vi "ScrollDataChange.vi"(0 "Actual Data":T1[](array[typedef]), 5 "Display Data":T1[](array[typedef]), 9 "Bounds  Of Picture":T3, 11 "Delta":i32) -> (4 "Actual Dataout":T1[](array[typedef]), 6 "Display Data out":T1[](array[typedef]), 8 "ScrollChange?":bool)   [LabVIEW 2014, in "SmartPalette.lvlib"]
uses:
  SmartPalette.lvlib
  Controls/Palette Data.ctl
  <vilib>/picture/picture.llb/imagedata.ctl
  <vilib>/Utility/miscctls.llb/LVBoundsTypeDef.ctl
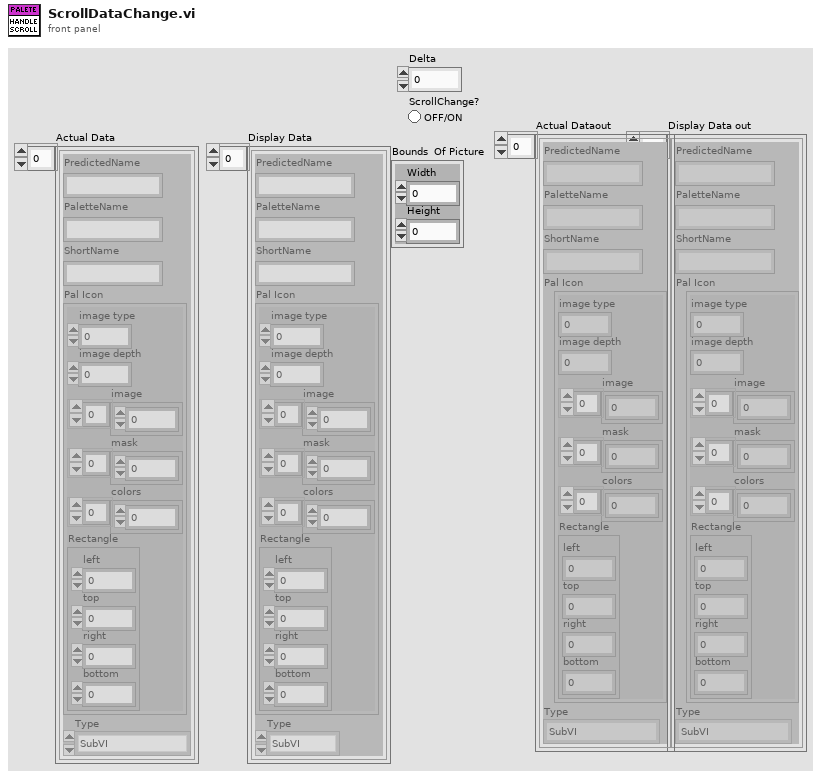
[diagram p1: front panel]
types:
  T1 = typedef "SmartPalette.lvlib/Palette Data.ctl" = cluster{"PredictedName":string, "PaletteName":string, "ShortName":string, "Pal Icon":T2, "Type":enum16{"SubVI", "VI Templtate", "Function"}}
  T2 = typedef "imagedata.ctl" = cluster{"image type":i32, "image depth":i32, "image":u8[], "mask":u8[], "colors":u32[], "Rectangle":cluster{"left":i16, "top":i16, "right":i16, "bottom":i16}}
  T3 = typedef "LVBoundsTypeDef.ctl" = cluster{"Width":u32, "Height":u32}
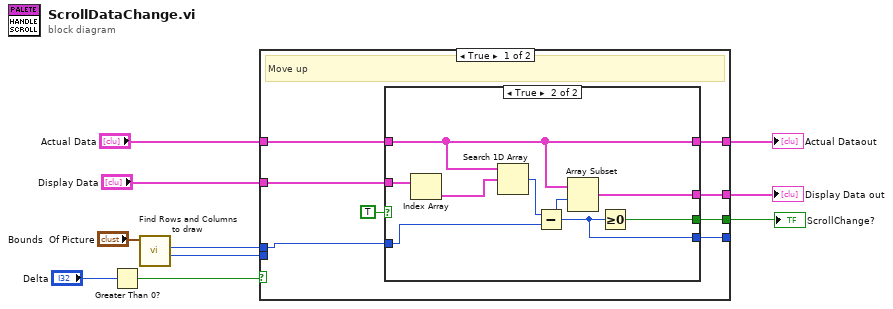
[diagram p0: block diagram]
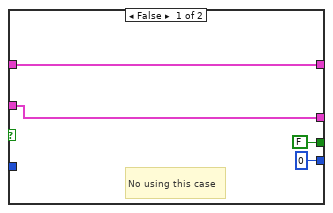
[diagram p2: hidden frame]
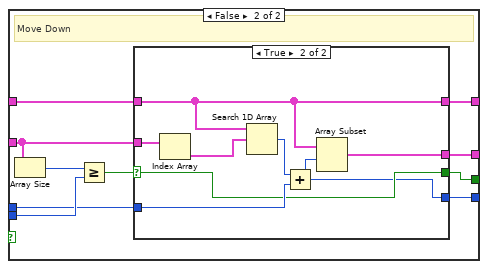
[diagram p3: hidden frame]
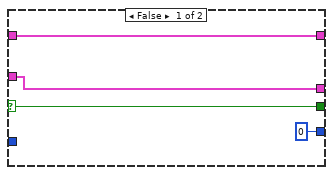
[diagram p4: hidden frame]
diagram:
  n1 = Greater Than 0?(x="Delta") -> (x > 0?=w9:bool)
  n2 = call "Find Rows and Columns to draw.vi"("Bounds  Of Picture"="Bounds  Of Picture") -> ("Total"=w1:u32, "Col"=w3:u32)  [unwired: 8 in, 1 out]
  n3 = case shown="True" w9 {
    tunnel: "Actual Data" -> [w18 w38]
    tunnel: "Display Data" -> [w17 w37]
    tunnel: [w16 w36] -> w5
    tunnel: [w15 w35] -> w4
    tunnel: [w13 w34] -> w7
    tunnel: w1 -> [_ w33]
    tunnel: w3 -> [w12 w32]
    tunnel: [w11 w31] -> _
    frame True {
      # "Move up"
      n4 = case shown="True" TRUE {
        tunnel: w12 -> [_ w27]
        tunnel: w18 -> [w22 w25]
        tunnel: w17 -> [w21 w30]
        tunnel: [w21 w26] -> w16
        tunnel: [w22 w25] -> w15
        tunnel: [FALSE w24] -> w13
        tunnel: [u32 0 w23] -> w11
        frame False {
          # "No using this case"
        }
        frame True {
          n5 = Index Array(array=w30) -> (element=w29:T1)  [unwired: 1 in]
          n6 = Search 1D Array(1D array=w25, element=w29) -> (index of element=w28:i32)  [unwired: 1 in]
          n7 = Subtract(x=w28, y=w27) -> (x-y=w23:u32)
          n8 = Array Subset(array=w25, index=w23) -> (w26:T1[])  [unwired: 1 in]
          n9 = Greater Or Equal To 0?(x=w23) -> (x >= 0?=w24:bool)
        }
      }
    }
    frame False {
      # "Move Down"
      n10 = Array Size(array=w37) -> (size(s)=w40:i32)
      n11 = Greater Or Equal?(x=w40, y=w33) -> (x >= y?=w39:bool)
      n12 = case shown="True" w39 {
        selector: w39 -> [w42 w46]
        tunnel: w32 -> [_ w49]
        tunnel: w38 -> [w44 w47]
        tunnel: w37 -> [w43 w52]
        tunnel: [w43 w48] -> w36
        tunnel: [w44 w47] -> w35
        tunnel: [w42 w46] -> w34
        tunnel: [u32 0 w45] -> w31
        frame False {
        }
        frame True {
          n13 = Index Array(array=w52) -> (element=w51:T1)  [unwired: 1 in]
          n14 = Search 1D Array(1D array=w47, element=w51) -> (index of element=w50:i32)  [unwired: 1 in]
          n15 = Add(x=w50, y=w49) -> (x+y=w45:u32)
          n16 = Array Subset(array=w47, index=w45) -> (w48:T1[])  [unwired: 1 in]
        }
      }
    }
  }
  "Display Data out" <- w5
  "Actual Dataout" <- w4
  "ScrollChange?" <- w7
